vi "Translator.Translate.Text.vi"(8 "error in":errorcluster, 10 "text":string="text") -> (0 "error out":errorcluster, 2 "translated text":string)   [LabVIEW 2019, in "Tools.lvlib"]
uses:
  Tools.lvlib
  Translator.Translate.Text.Buffer.FGV.Action.ctl
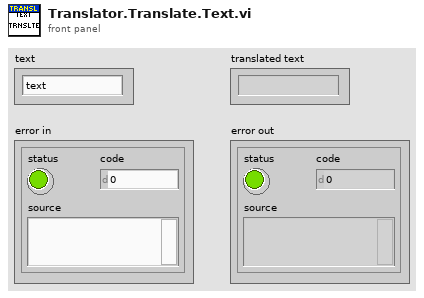
[diagram p1: front panel]
types:
  T1 = typedef "Tools.lvlib/Translator.Translate.Text.Buffer.FGV.Action.ctl" = enum16{"init", "get", "set"}
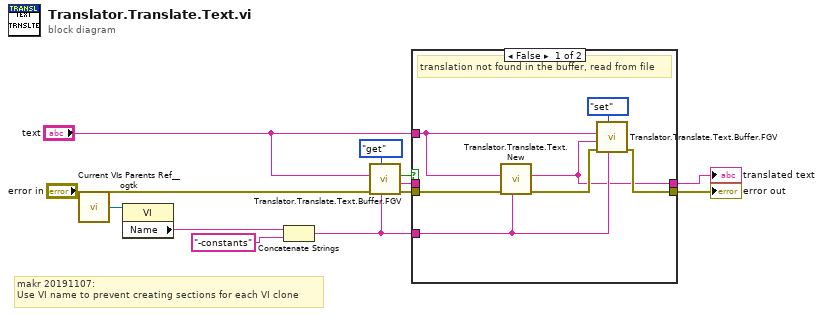
[diagram p0: block diagram]
diagram:
  # "makr 20191107:\nUse VI name to prevent creating sections for each VI clone"
  n1 = call <userlib>:"Current VIs Parents Ref__ogtk.vi"() -> ("Calling VI's Reference"=w1:refnum<vi>)  [unwired: 2 in]
  n2 = property class="VI"(reference=w1) -> ("Name"=w2:string)  [unwired: 1 in, 2 out]
  n3 = Concatenate Strings(w2, "-constants" ("string")) -> (w4:string)
  n4 = call "Translator.Translate.Text.Buffer.FGV.vi"("group"=w4, "action"=Translator.Translate.Text.Buffer.FGV.Action."get", "error in"="error in", "text"="text") -> ("error out"=w8:errorcluster, "translated"=w5:string, "found?"=w6:bool)  [unwired: 4 in, 1 out]
  n5 = case shown="False" w6 {
    tunnel: [w13 w21] -> w12
    tunnel: [w17 w20] -> w11
    tunnel: w8 -> [w19 w20]
    tunnel: w5 -> [_ w21]
    tunnel: w4 -> [w16 _]
    tunnel: "text" -> [w14 _]
    frame False {
      # "translation not found in the buffer, read from file"
      n6 = call "Translator.Translate.Text.New.vi"("group"=w16, "error in (no error)"=w19, "text"=w14) -> ("error out"=w18:errorcluster, "translated"=w13:string)  [unwired: 7 in]
      n7 = call "Translator.Translate.Text.Buffer.FGV.vi"("group"=w16, "action"=Translator.Translate.Text.Buffer.FGV.Action."set", "error in"=w18, "translated"=w13, "text"=w14) -> ("error out"=w17:errorcluster)  [unwired: 3 in, 3 out]
    }
    frame True {
      # "translation found in the buffer"
    }
  }
  "error out" <- w11
  "translated text" <- w12
